vi "CSMQ FGV Change Flag Name.vi"() -> (3 "Global-CSMQ FGV Change Flag":string)   [LabVIEW 2017, in "Communicable State Machine.lvlib"]
uses:
  Communicable State Machine.lvlib
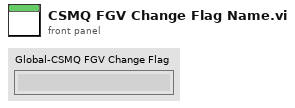
[diagram p1: front panel]
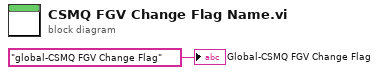
[diagram p0: block diagram]
diagram:
  "Global-CSMQ FGV Change Flag" <- "global-CSMQ FGV Change Flag" ("global-CSMQ FGV Change Flag")
